vi "Initialize.vi"(8 "error in (no error)":errorcluster, 10 "Resource Name in":T1, 11 "Loopback in":refnum<class "Loopback.lvclass">) -> (0 "error out":errorcluster, 3 "Loopback out":refnum<class "Loopback.lvclass">)   [LabVIEW 2015, in "Loopback.lvclass"]
uses:
  Loopback.lvclass
  <vilib>/userdefined/High Color/nirio_resource_hc.ctl
  Loopback.lvclass/Loopback.ctl
  <vilib>/FPGAPlugInAG/PXIe-7822R/niLvFpga_Open_PXIe-7822R.vi
  <vilib>/rvi/interface/common/dynamic/niFpgaDynamicAddResources.vi
  <vilib>/rvi/interface/nirviOpenFPGA/nirviOpenFPGA.xnode
  Loopback_FPGATarget_Loopback_3S22y2ZVP64.lvbitx
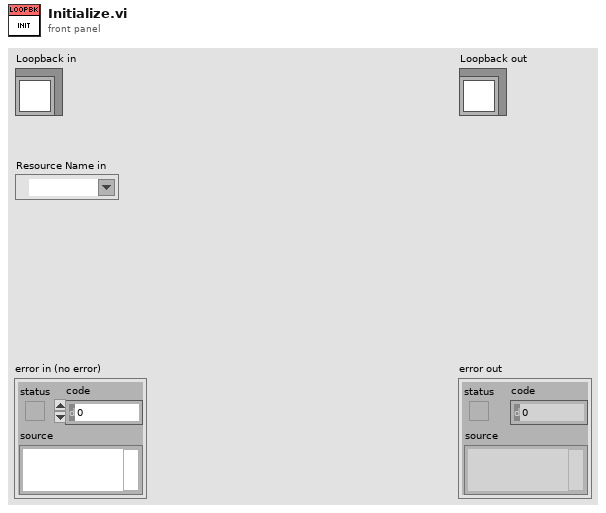
[diagram p1: front panel]
types:
  T1 = typedef "nirio_resource_hc.ctl" = tag
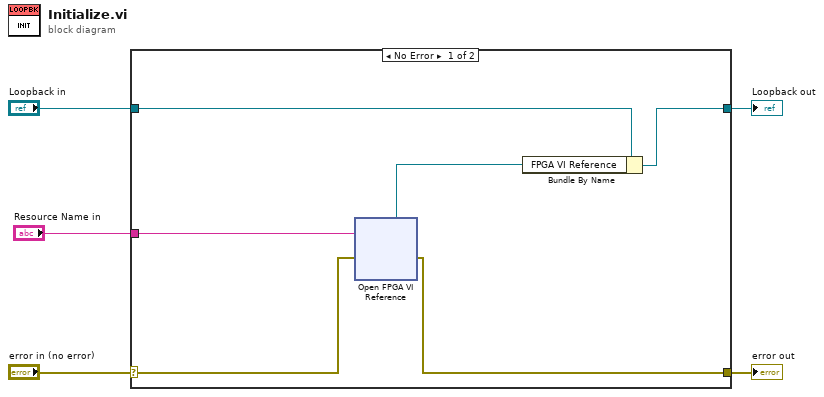
[diagram p0: block diagram]
diagram:
  n1 = case shown="No Error" "error in (no error)" {
    selector: "error in (no error)" -> [w8 w13]
    tunnel: [w7 w13] -> w4
    tunnel: [w10 w12] -> w2
    tunnel: "Loopback in" -> [w11 w12]
    tunnel: "Resource Name in" -> [w9 _]
    frame No Error {
      n2 = xnode "Open FPGA VI Reference"("error in"=w8, "resource name"=w9) -> ("FPGA VI Reference Out"=w6:refnum<k20>, "error out"=w7:errorcluster)
      n3 = Bundle By Name(cluster=w11, "FPGA VI Reference"=w6) -> (w10:refnum<class "Loopback.lvclass">)
    }
    frame Error {
    }
  }
  "error out" <- w4
  "Loopback out" <- w2
